vi "EXA_getEvent_Heartbeat.vi"(8 "error in (no error)":errorcluster, 11 "logevent_Heartbeat_Ctl":T1) -> (0 "error out":errorcluster, 2 "function return":i32, 3 "logevent_Heartbeat_Ctl out":T1)   [LabVIEW 2016, in "SALLV_EXA.lvlib"]
doc: "int EXA_shm_getEvent_HeartbeatLV(EXA_logevent_HeartbeatLV *logevent_Heartbeat_Ctl );"
uses:
  SALLV_EXA.lvlib
  DataTypes/logevent_Heartbeat.ctl
  SALLV_EXA.so
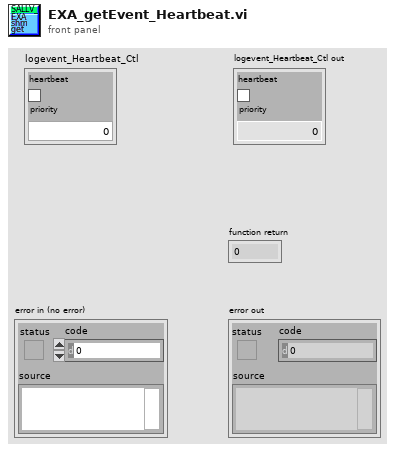
[diagram p1: front panel]
types:
  T1 = typedef "SALLV_EXA.lvlib/logevent_Heartbeat.ctl" = cluster{"heartbeat":bool, "priority":i32}
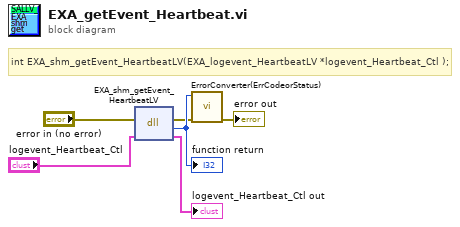
[diagram p0: block diagram]
diagram:
  # "int EXA_shm_getEvent_HeartbeatLV(EXA_logevent_HeartbeatLV *logevent_Heartbeat_Ctl );"
  n1 = dll-call lib="home/andres/Desktop/ts_sallv_EXA2/SALLV_EXA.*" fn="EXA_shm_getEvent_HeartbeatLV"(error in="error in (no error)", "logevent_Heartbeat_Ctl"="logevent_Heartbeat_Ctl") -> (error out=w2:errorcluster, w6:i32, "logevent_Heartbeat_Ctl"=→"logevent_Heartbeat_Ctl out":T1)  [unwired: 2 in, 1 out]
  "function return" <- w6
  n2 = call "ErrorConverter(ErrCodeorStatus).vi"("error in (no error)"=w2, "error code"=w6) -> ("error out"=→"error out":errorcluster)  [unwired: 9 in]
